vi "Configure Port Extension.vi"(5 "Port 1 (1)":i32=1, 7 "Channel (1)":i32=1, 8 "error in (no error)":errorcluster, 9 "Correction Value (0.0)":dbl format="%.2f", 10 "Port Extension State (F: Disabled)":bool, 11 "VISA resource name":refnum<visa-resource-name>) -> (0 "error out":errorcluster, 3 "VISA resource name out":refnum<visa-resource-name>)   [LabVIEW 2012, in "Tektronix TTR500 Series.lvlib"]
doc: "This function configure port extension settings."
uses:
  <instrlib>/Tektronix TTR500 Series/Tektronix TTR500 Series.lvlib
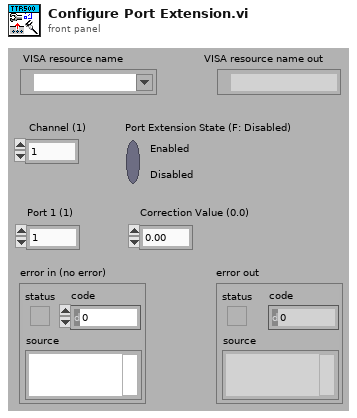
[diagram p1: front panel]
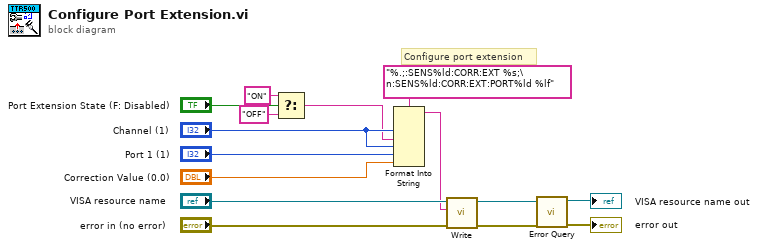
[diagram p0: block diagram]
diagram:
  # "Configure port extension"
  n1 = Select(t="ON", s="Port Extension State (F: Disabled)", f="OFF") -> (s? t:f=w7:string)
  n2 = Format Into String(format string="%.;:SENS%ld:CORR:EXT %s;\n:SENS%ld:CORR:EXT:PORT%ld %lf", "Channel (1)", w7, "Channel (1)", "Port 1 (1)", "Correction Value (0.0)") -> (resulting string=w12:string)  [unwired: 2 in, 1 out]
  n3 = call <instrlib>:"Write.vi"("error in (no error)"="error in (no error)", "String ()"=w12, "VISA resource name"="VISA resource name") -> ("error out"=w3:errorcluster, "VISA resource name out"=w4:refnum<visa-resource-name>)  [unwired: 6 in, 1 out]
  n4 = call <instrlib>:"Error Query.vi"("error in (no error)"=w3, "VISA resource name"=w4) -> ("error out"=→"error out":errorcluster, "VISA resource name out"=→"VISA resource name out":refnum<visa-resource-name>)  [unwired: 6 in, 2 out]
